vi "Get - Boolean.vi"(7 "PV name":string, 8 "error in (no error)":errorcluster, 9 "timeout":dbl[unit]=1.0, 10 "default":bool, 11 "Client in":refnum<class "Client.lvclass">) -> (0 "error out":errorcluster, 1 "timed out?":bool, 2 "value":bool, 3 "Client out":refnum<class "Client.lvclass">, 4 "timestamp":timestamp)   [LabVIEW 2020, in "PV Access.lvlib" / "PVA Client.lvlib" / "Client.lvclass"]
uses:
  Client.lvclass
  Client.lvclass/Client.ctl
  67d96ea5-d90b-48b4-901c-0faecaf72cae.vi
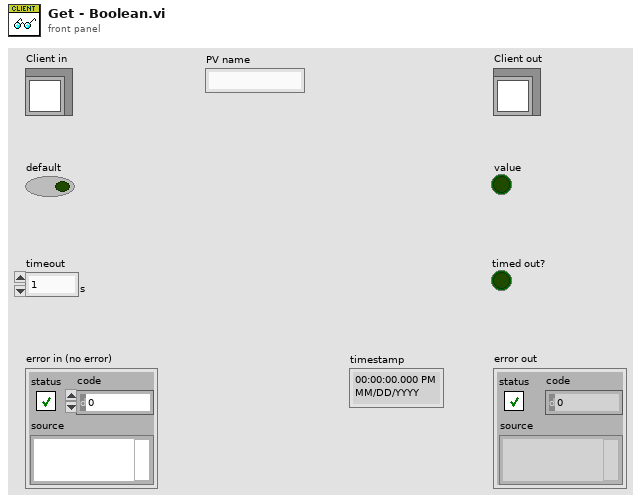
[diagram p1: front panel]
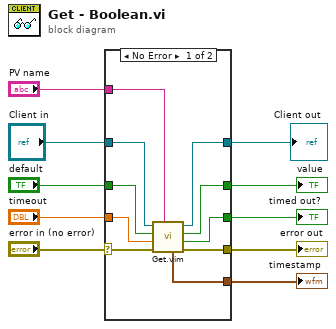
[diagram p0: block diagram]
diagram:
  n1 = case shown="No Error" "error in (no error)" {
    selector: "error in (no error)" -> [w13 w23]
    tunnel: [w12 w23] -> w9
    tunnel: [w14 w22] -> w7
    tunnel: "Client in" -> [w15 w22]
    tunnel: "default" -> [w20 w21]
    tunnel: [w19 w21] -> w5
    tunnel: "timeout" -> [w18 _]
    tunnel: [w17 _] -> w3
    tunnel: "PV name" -> [w16 _]
    tunnel: [w11 _] -> w1
    frame No Error {
      n2 = call "Get.vim"("PV name"=w16, "error in"=w13, "timeout"=w18, "data type"=w20, "Client in"=w15) -> ("error out"=w12:errorcluster, "timed out?"=w17:bool, "value"=w19:bool, "Client out"=w14:refnum<class "Client.lvclass">, "timestamp"=w11:timestamp)  [unwired: 2 in]
    }
    frame Error {
    }
  }
  "error out" <- w9
  "Client out" <- w7
  "value" <- w5
  "timed out?" <- w3
  "timestamp" <- w1
